vi "Register.vi"(6 "Save Parameters":variant, 8 "error in (no error)":errorcluster, 9 "Name":string, 10 "GetData Message":T1, 11 "StorageService in":refnum<class "StorageService.lvclass">) -> (0 "error out":errorcluster, 3 "StorageService out":refnum<class "StorageService.lvclass">)   [LabVIEW 2014, in "StorageService.lvclass"]
uses:
  StorageService.lvclass
  <vilib>/ActorFramework/Message Enqueuer/Message Enqueuer.lvclass
  Model/ReplayData Msg/ReplayData Msg.lvclass
  StorageService.lvclass/StorageService.ctl
  RegisteredObject.ctl
  Model/Data/AbstractData/AbstractData.lvclass
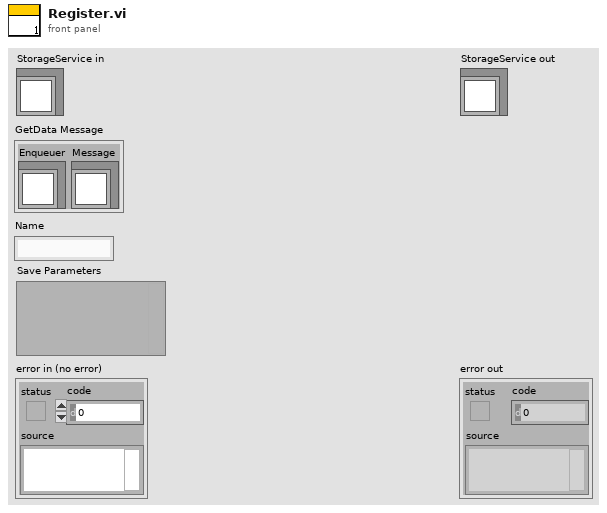
[diagram p1: front panel]
types:
  T1 = cluster{"Enqueuer":refnum<class "Message Enqueuer.lvclass">, "Message":refnum<class "ReplayData Msg.lvclass">}
  T2 = cluster{"Data":refnum<class "AbstractData.lvclass">, "Parameter":refnum<class "AbstractData.lvclass">}
  T3 = typedef "StorageService.lvclass/RegisteredObject.ctl" = cluster{"Name":string, "Is Acquired":bool, "Queue":refnum<queue>, "Message To Send":cluster{"Enqueuer":refnum<class "Message Enqueuer.lvclass">, "Message":refnum<class "ReplayData Msg.lvclass">}, "Save Parameters":variant}
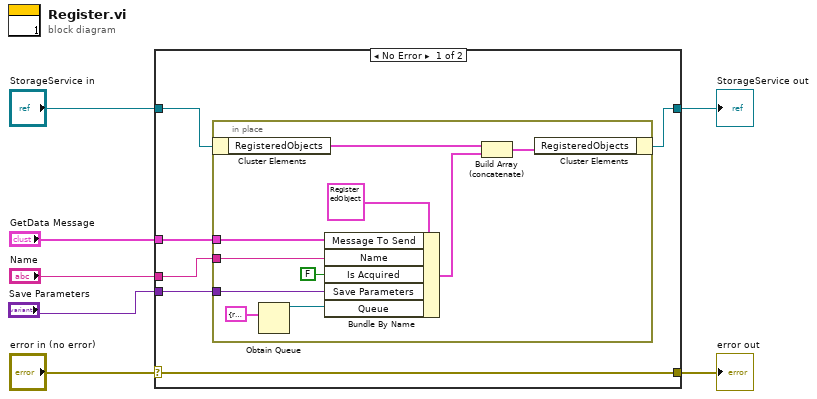
[diagram p0: block diagram]
diagram:
  n1 = case shown="No Error" "error in (no error)" {
    selector: "error in (no error)" -> [w13 w25]
    tunnel: [w13 w25] -> w6
    tunnel: [w9 w24] -> w4
    tunnel: "StorageService in" -> [w10 w24]
    tunnel: "Name" -> [w11 _]
    tunnel: "GetData Message" -> [w12 _]
    tunnel: "Save Parameters" -> [w8 _]
    frame No Error {
      n2 = in-place {
        in-place-border: w12 -> [w18]
        in-place-border: w11 -> [w21]
        in-place-border: w8 -> [w16]
        n3 = in-place-cluster #1(w10) -> ("RegisteredObjects"=w23:T3[])
        n4 = Obtain Queue(element data type=T2 {"Data"=refnum, "Parameter"=refnum} ("element")) -> (queue out=w14:refnum<queue>)  [unwired: 4 in, 2 out]
        n5 = Bundle By Name(cluster=T3 {"Name"="", "Is Acquired"=FALSE, "Queue"=refnum, "Message To Send"={"Enqueuer"=refnum, "Message"=refnum}, "Save Parameters"=variant(bool FALSE)} ("Cluster"), "Message To Send"=w18, "Name"=w21, "Is Acquired"=FALSE, "Save Parameters"=w16, "Queue"=w14) -> (w22:T3)
        n6 = Build Array (concatenate)(w23, w22) -> (w19:T3[])
        n7 = in-place-cluster #1("RegisteredObjects"=w19) -> (w9:refnum<class "StorageService.lvclass">)
      }
    }
    frame Error {
    }
  }
  "error out" <- w6
  "StorageService out" <- w4
